vi "Autonomous Independent.vi"   [LabVIEW 2016]
doc: "This VI is called when autonomous begins, and will automatically be terminated when autonomous ends. You can carry out timed or sensor driven robot movement independently without needing to return to the caller."
uses:
  <vilib>/Rock Robotics/WPI/Solenoid/WPI_SolenoidValue.ctl
  <vilib>/Rock Robotics/WPI/DriverStation/WPI_DriverStationAllianceInfo.ctl
  <vilib>/Rock Robotics/Network Tables/NT Read Number.vi
  <vilib>/Rock Robotics/WPI/Solenoid/WPI_SolenoidSetEnum.vi
  Robot Global Data.vi
panel:
  # "Be sure to right-click and choose Data Operations>>Make Current Value default if you want to save the array values with the VI"
types:
  T1 = typedef "WPI_DriverStationAllianceInfo.ctl" = enum16{"Red", "Blue", "Invalid"}
  T2 = typedef "WPI_SolenoidValue.ctl" = enum16{"Off", "On", "Forward", "Reverse"}
  T3 = typedef "WPI_MotorControlDeviceRef.ctl" = cluster{"DeviceStatus":errorcluster, "Type":T4, "PWM":cluster{"PWM Channel":T5, "DeadBand":T6}, "CAN":cluster{"Device Number":u8, "SetOutput VI Ref":variant, "GetOutput VI Ref":variant, "Enable VI Ref":variant, "Disable VI Ref":variant, "Data":variant}, "Invert":bool}
  T4 = typedef "WPI_MotorControlType.ctl" = enum16{"PWM", "CAN"}
  T5 = typedef "FPGA_DIOPWMChannel.ctl" = enum8{"PWM 0", "PWM 1", "PWM 2", "PWM 3", "PWM 4", "PWM 5", "PWM 6", "PWM 7", "PWM 8", "PWM 9", "PWM MXP 0", "PWM MXP 1", "PWM MXP 2", "PWM MXP 3", "PWM MXP 4", "PWM MXP 5", "PWM MXP 6", "PWM MXP 7", "PWM MXP 8", "PWM MXP 9", "Invalid"}
  T6 = typedef "WPI_PWMDeadband.ctl" = cluster{"Name":string, "maxPositivePwm":i32, "minPositivePwm":i32, "centerPwm":i32, "maxNegativePwm":i32, "minNegativePwm":i32, "angularRange":u16}
  T7 = typedef "WPI_SolenoidDevRef.ctl" = cluster{"DevStatus":errorcluster, "Pneumatics Control Module":u8, "Forward Solenoid Channel":T8, "Reverse Solenoid Channel":T8}
  T8 = typedef "WPI_SolenoidChannel.ctl" = enum8{"Solenoid 0", "Solenoid 1", "Solenoid 2", "Solenoid 3", "Solenoid 4", "Solenoid 5", "Solenoid 6", "Solenoid 7", "Invalid"}
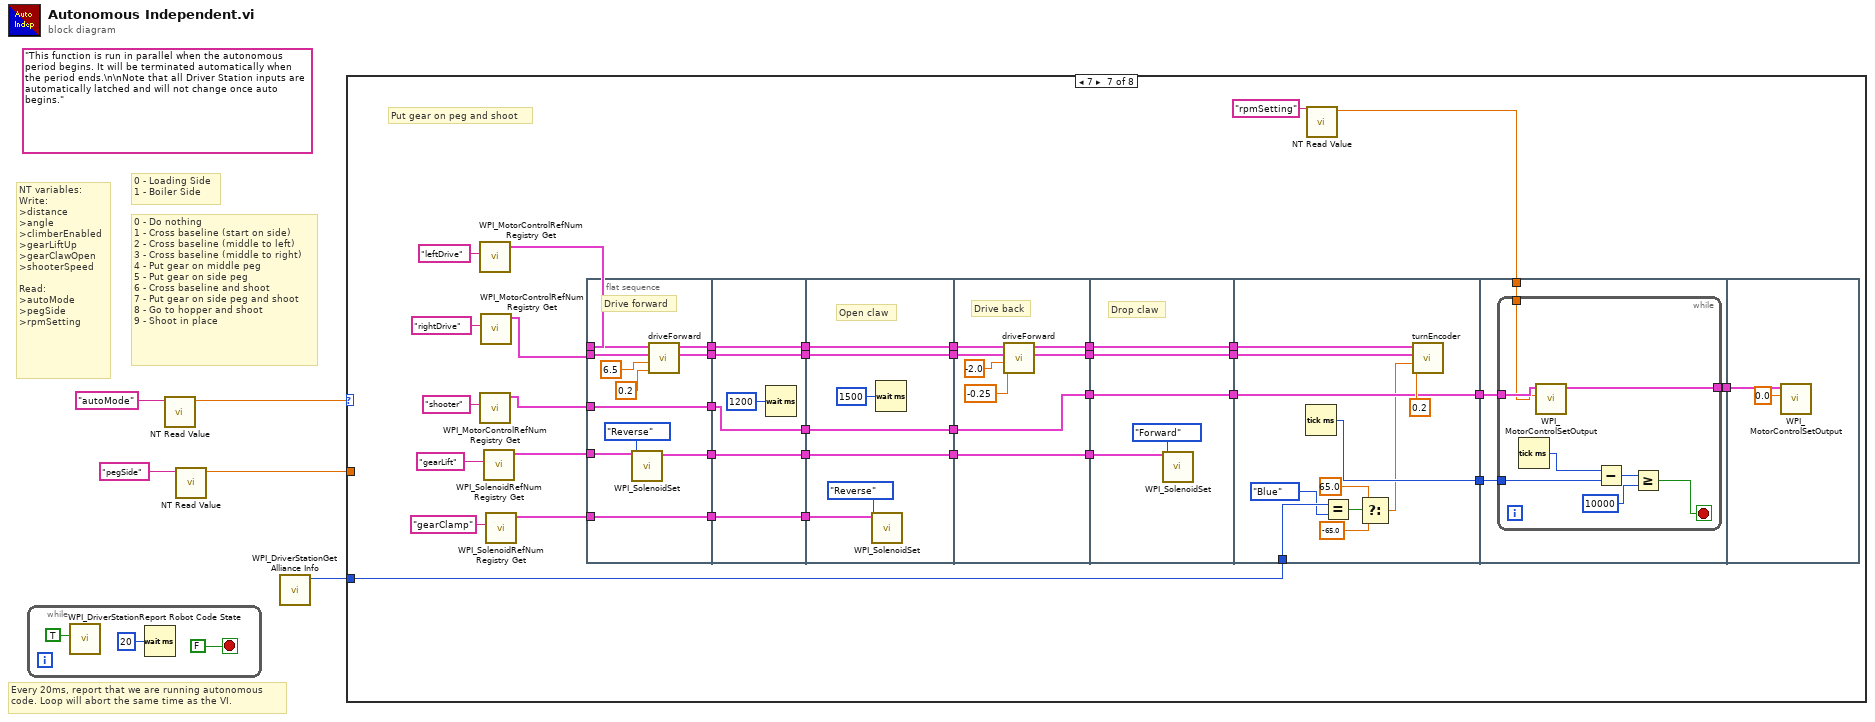
[diagram p0: block diagram]
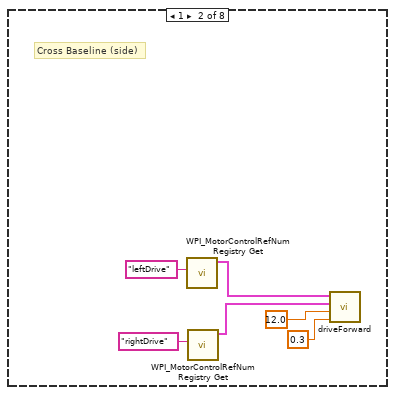
[diagram p3: hidden frame]
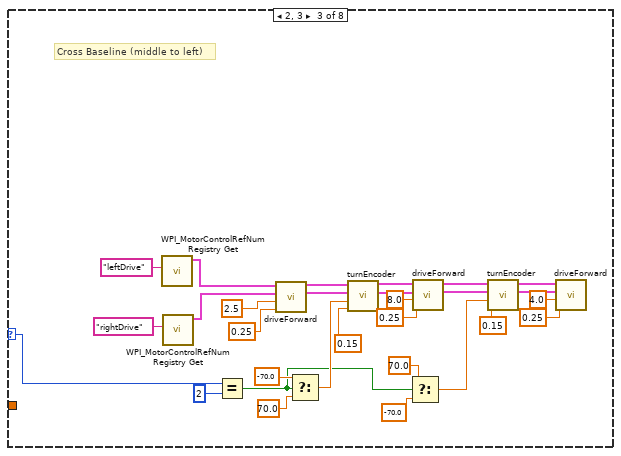
[diagram p4: hidden frame]
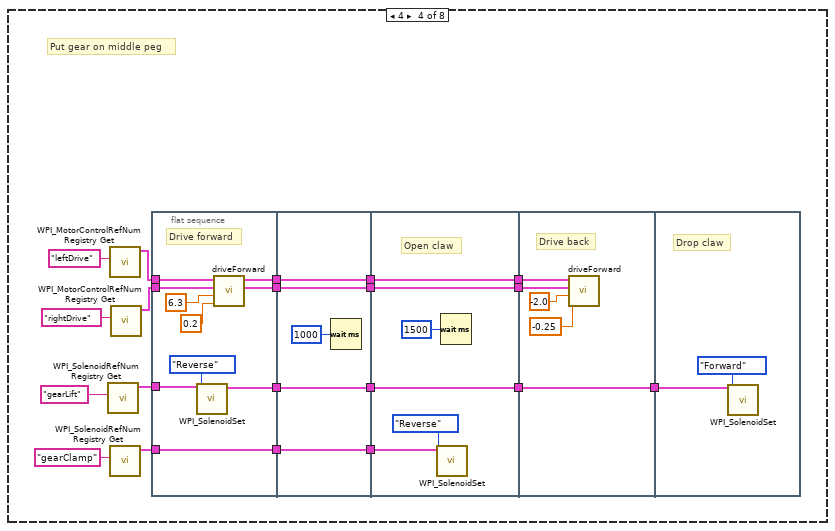
[diagram p5: hidden frame]
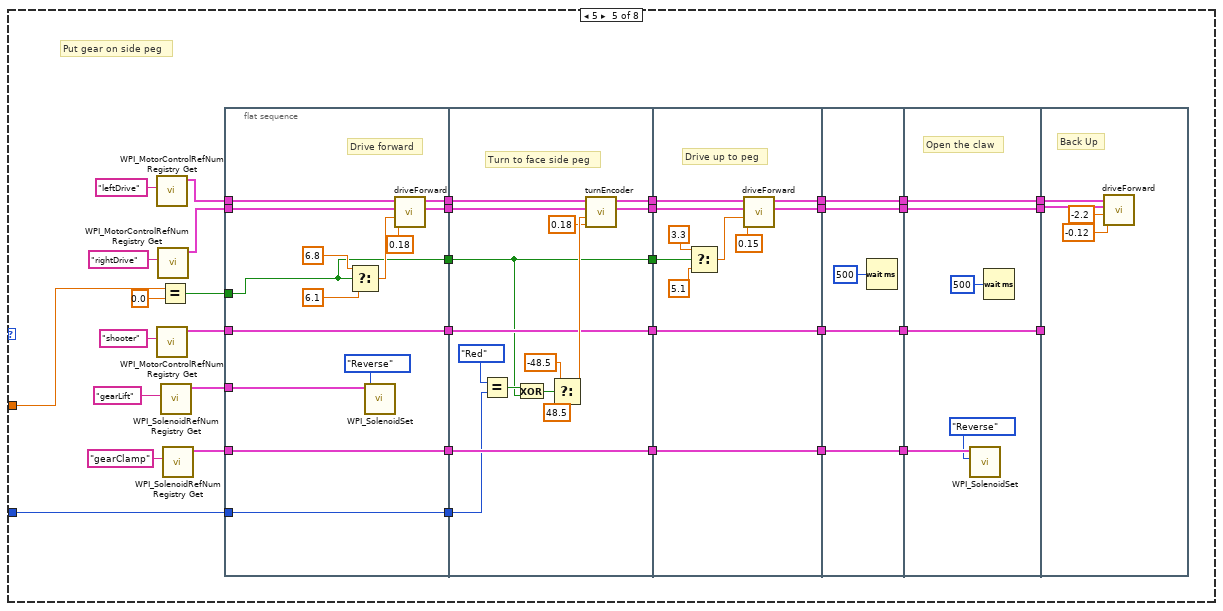
[diagram p6: hidden frame]
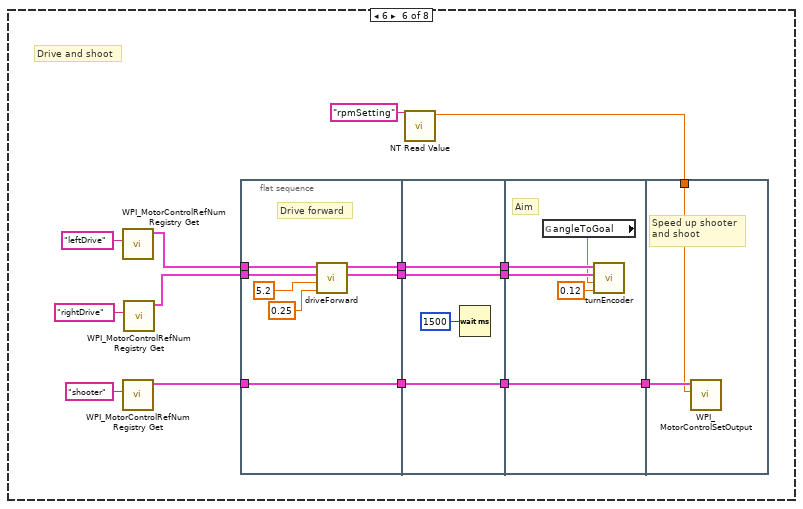
[diagram p7: hidden frame]
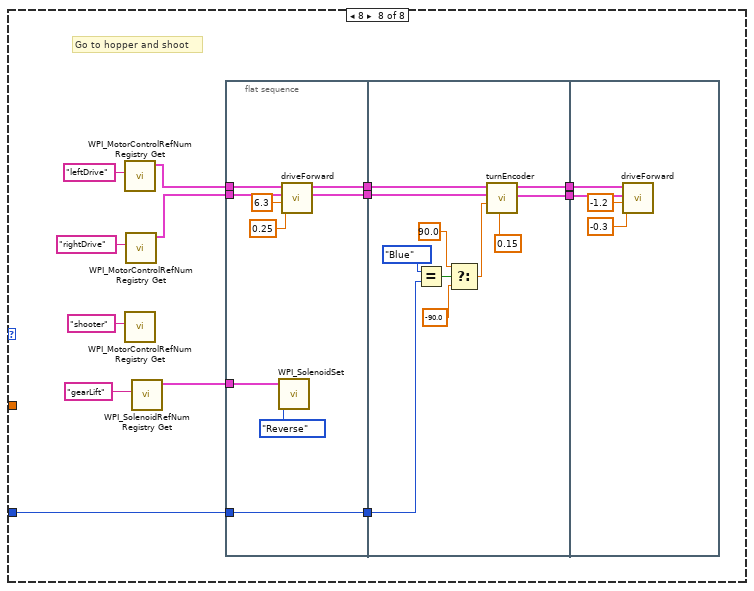
[diagram p8: hidden frame]
diagram:
  (unwired) "This function is run in parallel when the autonomous period begins. It will be terminated automatically when the period ends.\n\nNote that all Driver Station inputs are automatically latched and will not change once auto begins."
  # "0 - Loading Side\n1 - Boiler Side"
  # "NT variables:\nWrite:\n>distance\n>angle\n>climberEnabled\n>gearLiftUp\n>gearClawOpen\n>shooterSpeed\n\nRead:\n>autoMode\n>pegSide\n>rpmSetting"
  # "0 - Do nothing\n1 - Cross baseline (start on side)\n2 - Cross baseline (middle to left)\n3 - Cross baseline (middle to right)\n4 - Put gear on middle peg\n5 - Put gear on side peg\n6 - Cross baseline and shoot\n7 - Put gear on side peg and shoot\n8 - Go to hopper and shoot\n9 - Shoot in place"
  # "Every 20ms, report that we are running autonomous\ncode. Loop will abort the same time as the VI."
  n1 = while {
    stop <- FALSE stop-if-true
    n2 = call <vilib>:"WPI_DriverStationReport Robot Code State.vi"("Autonomous"=TRUE) -> ()  [unwired: 10 in, 1 out]
    n3 = Wait (ms)(milliseconds to wait=u32 20) -> ()  [unwired: 1 out]
  }
  n4 = call-poly <vilib>:"NT Read Value.vi"("Name"="autoMode") -> ("Numeric"=w3:dbl)  [unwired: 9 in, 1 out]
  n5 = call-poly <vilib>:"NT Read Value.vi"("Name"="pegSide") -> ("Numeric"=w1:dbl)  [unwired: 9 in, 1 out]
  n6 = call <vilib>:"WPI_DriverStationGet Alliance Info.vi"() -> ("Alliance"=w4:T1)  [unwired: 11 out]
  n7 = case shown="7" w3 {
    selector: w3 -> [_ _ w20 _ _ _ _ _]
    tunnel: w4 -> [_ _ _ _ w105 _ w216 w318]
    tunnel: w1 -> [_ _ _ _ w103 _ _ _]
    frame 0, Default {
      # "Do nothing"
    }
    frame 1 {
      # "Cross Baseline (side)"
      n8 = call <vilib>:"WPI_MotorControlRefNum Registry Get.vi"("refnum name"="leftDrive") -> ("MotorControlDevRef"=w12:T3)  [unwired: 9 in, 1 out]
      n9 = call <vilib>:"WPI_MotorControlRefNum Registry Get.vi"("refnum name"="rightDrive") -> ("MotorControlDevRef"=w11:T3)  [unwired: 9 in, 1 out]
      n10 = call "driveForward.vi"("speed (%)"=0.3, "distance (ft)"=12.0, "rightMotor"=w11, "leftMotor"=w12) -> ()  [unwired: 6 in, 2 out]
    }
    frame 2, 3 {
      # "Cross Baseline (middle to left)"
      n11 = call <vilib>:"WPI_MotorControlRefNum Registry Get.vi"("refnum name"="leftDrive") -> ("MotorControlDevRef"=w41:T3)  [unwired: 9 in, 1 out]
      n12 = call <vilib>:"WPI_MotorControlRefNum Registry Get.vi"("refnum name"="rightDrive") -> ("MotorControlDevRef"=w40:T3)  [unwired: 9 in, 1 out]
      n13 = Equal?(x=w20, y=2) -> (x = y?=w15:bool)
      n14 = call "driveForward.vi"("speed (%)"=0.25, "distance (ft)"=2.5, "rightMotor"=w40, "leftMotor"=w41) -> ("rightMotor"=w36:T3, "leftMotor"=w37:T3)  [unwired: 6 in]
      n15 = Select(t=-70.0 ("angle (ccw)"), s=w15, f=70.0 ("angle (ccw)")) -> (s? t:f=w22:dbl)
      n16 = call "turnEncoder.vi"("speed (%)"=0.15, "angle (right)"=w22, "rightMotor"=w36, "leftMotor"=w37) -> ("rightMotor"=w33:T3, "leftMotor"=w34:T3)  [unwired: 6 in]
      n17 = Select(t=70.0 ("angle (ccw)"), s=w15, f=-70.0) -> (s? t:f=w17:dbl)
      n18 = call "driveForward.vi"("speed (%)"=0.25, "distance (ft)"=8.0, "rightMotor"=w33, "leftMotor"=w34) -> ("rightMotor"=w29:T3, "leftMotor"=w30:T3)  [unwired: 6 in]
      n19 = call "turnEncoder.vi"("speed (%)"=0.15, "angle (right)"=w17, "rightMotor"=w29, "leftMotor"=w30) -> ("rightMotor"=w26:T3, "leftMotor"=w27:T3)  [unwired: 6 in]
      n20 = call "driveForward.vi"("speed (%)"=0.25, "distance (ft)"=4.0, "rightMotor"=w26, "leftMotor"=w27) -> ()  [unwired: 6 in, 2 out]
    }
    frame 4 {
      # "Put gear on middle peg"
      n21 = call <vilib>:"WPI_SolenoidRefNum Registry Get.vi"("refnum name"="gearLift") -> ("SolenoidDevRef"=w57:T7)  [unwired: 9 in, 1 out]
      n22 = call <vilib>:"WPI_MotorControlRefNum Registry Get.vi"("refnum name"="leftDrive") -> ("MotorControlDevRef"=w61:T3)  [unwired: 9 in, 1 out]
      n23 = call <vilib>:"WPI_SolenoidRefNum Registry Get.vi"("refnum name"="gearClamp") -> ("SolenoidDevRef"=w56:T7)  [unwired: 9 in, 1 out]
      n24 = call <vilib>:"WPI_MotorControlRefNum Registry Get.vi"("refnum name"="rightDrive") -> ("MotorControlDevRef"=w60:T3)  [unwired: 9 in, 1 out]
      n25 = flat-sequence {
        tunnel: w61 -> [w73]
        tunnel: w60 -> [w72]
        tunnel: w57 -> [w69]
        tunnel: [w67] -> w51
        tunnel: w56 -> [w67]
        tunnel: [w66] -> w49
        tunnel: [w65] -> w47
        tunnel: [w64] -> w45
        tunnel: w51 -> [w78]
        tunnel: [w78] -> w50
        tunnel: w49 -> [w77]
        tunnel: [w77] -> w48
        tunnel: w47 -> [w76]
        tunnel: [w76] -> w46
        tunnel: w45 -> [w75]
        tunnel: [w75] -> w44
        tunnel: w50 -> [w84]
        tunnel: [w82] -> w55
        tunnel: w48 -> [w82]
        tunnel: [w81] -> w54
        tunnel: w46 -> [w81]
        tunnel: [w80] -> w52
        tunnel: w44 -> [w80]
        tunnel: w55 -> [w89]
        tunnel: w54 -> [w88]
        tunnel: [w85] -> w53
        tunnel: w52 -> [w85]
        tunnel: w53 -> [w90]
        frame #0 {
          # "Drive forward"
          n26 = call-poly <vilib>:"WPI_SolenoidSet.vi"("Value"=WPI_SolenoidValue."Reverse", "SolenoidDevRef"=w69) -> ("SolenoidDevRef"=w64:T7)  [unwired: 8 in, 1 out]
          n27 = call "driveForward.vi"("speed (%)"=0.2, "distance (ft)"=6.3, "rightMotor"=w72, "leftMotor"=w73) -> ("rightMotor"=w65:T3, "leftMotor"=w66:T3)  [unwired: 6 in]
        }
        frame #1 {
          n28 = Wait (ms)(milliseconds to wait=u32 1000) -> ()  [unwired: 1 out]
        }
        frame #2 {
          # "Open claw"
          n29 = call-poly <vilib>:"WPI_SolenoidSet.vi"("Value"=WPI_SolenoidValue."Reverse", "SolenoidDevRef"=w84) -> ()  [unwired: 8 in, 2 out]
          n30 = Wait (ms)(milliseconds to wait=u32 1500) -> ()  [unwired: 1 out]
        }
        frame #3 {
          # "Drive back"
          n31 = call "driveForward.vi"("speed (%)"=-0.25, "distance (ft)"=-2.0, "rightMotor"=w88, "leftMotor"=w89) -> ()  [unwired: 6 in, 2 out]
        }
        frame #4 {
          # "Drop claw"
          n32 = call-poly <vilib>:"WPI_SolenoidSet.vi"("Value"=WPI_SolenoidValue."Forward", "SolenoidDevRef"=w90) -> ()  [unwired: 8 in, 2 out]
        }
      }
    }
    frame 5 {
      # "Put gear on side peg"
      n33 = call <vilib>:"WPI_MotorControlRefNum Registry Get.vi"("refnum name"="leftDrive") -> ("MotorControlDevRef"=w110:T3)  [unwired: 9 in, 1 out]
      n34 = call <vilib>:"WPI_MotorControlRefNum Registry Get.vi"("refnum name"="shooter") -> ("MotorControlDevRef"=w106:T3)  [unwired: 9 in, 1 out]
      n35 = call <vilib>:"WPI_MotorControlRefNum Registry Get.vi"("refnum name"="rightDrive") -> ("MotorControlDevRef"=w109:T3)  [unwired: 9 in, 1 out]
      n36 = Equal?(x=w103, y=0.0) -> (x = y?=w102:bool)
      n37 = call <vilib>:"WPI_SolenoidRefNum Registry Get.vi"("refnum name"="gearLift") -> ("SolenoidDevRef"=w108:T7)  [unwired: 9 in, 1 out]
      n38 = call <vilib>:"WPI_SolenoidRefNum Registry Get.vi"("refnum name"="gearClamp") -> ("SolenoidDevRef"=w107:T7)  [unwired: 9 in, 1 out]
      n39 = flat-sequence {
        tunnel: w110 -> [w141]
        tunnel: w109 -> [w140]
        tunnel: w105 -> [w138]
        tunnel: [w138] -> w127
        tunnel: [w137] -> w126
        tunnel: [w136] -> w125
        tunnel: w108 -> [w135]
        tunnel: [w133] -> w124
        tunnel: w107 -> [w133]
        tunnel: [w132] -> w123
        tunnel: w106 -> [w132]
        tunnel: w102 -> [w128]
        tunnel: [w128] -> w101
        tunnel: w127 -> [w142]
        tunnel: w126 -> [w153]
        tunnel: w125 -> [w152]
        tunnel: [w149] -> w122
        tunnel: [w148] -> w121
        tunnel: [w147] -> w120
        tunnel: w124 -> [w147]
        tunnel: w123 -> [w146]
        tunnel: [w146] -> w119
        tunnel: w101 -> [w143]
        tunnel: [w143] -> w100
        tunnel: w122 -> [w166]
        tunnel: w121 -> [w165]
        tunnel: [w164] -> w99
        tunnel: w120 -> [w164]
        tunnel: [w163] -> w97
        tunnel: [w162] -> w95
        tunnel: [w161] -> w93
        tunnel: w119 -> [w161]
        tunnel: w100 -> [w158]
        tunnel: w99 -> [w172]
        tunnel: [w172] -> w98
        tunnel: w97 -> [w171]
        tunnel: [w171] -> w96
        tunnel: w95 -> [w170]
        tunnel: [w170] -> w94
        tunnel: w93 -> [w169]
        tunnel: [w169] -> w92
        tunnel: w98 -> [w178]
        tunnel: [w176] -> w118
        tunnel: w96 -> [w176]
        tunnel: w94 -> [w175]
        tunnel: [w175] -> w117
        tunnel: [w174] -> w116
        tunnel: w92 -> [w174]
        tunnel: w118 -> [w182]
        tunnel: w117 -> [w181]
        tunnel: w116 -> [_]
        frame #0 {
          # "Drive forward"
          n40 = Select(t=6.8 ("distance (ft)"), s=w128, f=6.1) -> (s? t:f=w131:dbl)
          n41 = call-poly <vilib>:"WPI_SolenoidSet.vi"("Value"=WPI_SolenoidValue."Reverse", "SolenoidDevRef"=w135) -> ()  [unwired: 8 in, 2 out]
          n42 = call "driveForward.vi"("speed (%)"=0.18, "distance (ft)"=w131, "rightMotor"=w140, "leftMotor"=w141) -> ("rightMotor"=w136:T3, "leftMotor"=w137:T3)  [unwired: 6 in]
        }
        frame #1 {
          # "Turn to face side peg"
          n43 = Equal?(x=WPI_DriverStationAllianceInfo."Red" ("Alliance"), y=w142) -> (x = y?=w145:bool)
          n44 = Exclusive Or(1:w143, 2:w145) -> (0:w144:bool)
          n45 = Select(t=-48.5, s=w144, f=48.5) -> (s? t:f=w151:dbl)
          n46 = call "turnEncoder.vi"("speed (%)"=0.18, "angle (right)"=w151, "rightMotor"=w152, "leftMotor"=w153) -> ("rightMotor"=w148:T3, "leftMotor"=w149:T3)  [unwired: 6 in]
        }
        frame #2 {
          # "Drive up to peg"
          n47 = Select(t=3.3 ("distance (ft)"), s=w158, f=5.1) -> (s? t:f=w159:dbl)
          n48 = call "driveForward.vi"("speed (%)"=0.15, "distance (ft)"=w159, "rightMotor"=w165, "leftMotor"=w166) -> ("rightMotor"=w162:T3, "leftMotor"=w163:T3)  [unwired: 6 in]
        }
        frame #3 {
          n49 = Wait (ms)(milliseconds to wait=u32 500) -> ()  [unwired: 1 out]
        }
        frame #4 {
          # "Open the claw"
          n50 = call-poly <vilib>:"WPI_SolenoidSet.vi"("Value"=WPI_SolenoidValue."Reverse", "SolenoidDevRef"=w178) -> ()  [unwired: 8 in, 2 out]
          n51 = Wait (ms)(milliseconds to wait=u32 500) -> ()  [unwired: 1 out]
        }
        frame #5 {
          # "Back Up"
          n52 = call "driveForward.vi"("speed (%)"=-0.12, "distance (ft)"=-2.2, "rightMotor"=w181, "leftMotor"=w182) -> ()  [unwired: 6 in, 2 out]
        }
      }
    }
    frame 6 {
      # "Drive and shoot"
      n53 = call <vilib>:"WPI_MotorControlRefNum Registry Get.vi"("refnum name"="leftDrive") -> ("MotorControlDevRef"=w195:T3)  [unwired: 9 in, 1 out]
      n54 = call <vilib>:"WPI_MotorControlRefNum Registry Get.vi"("refnum name"="shooter") -> ("MotorControlDevRef"=w190:T3)  [unwired: 9 in, 1 out]
      n55 = call <vilib>:"WPI_MotorControlRefNum Registry Get.vi"("refnum name"="rightDrive") -> ("MotorControlDevRef"=w194:T3)  [unwired: 9 in, 1 out]
      n56 = flat-sequence {
        tunnel: w195 -> [w204]
        tunnel: w194 -> [w203]
        tunnel: [w200] -> w188
        tunnel: [w199] -> w186
        tunnel: [w198] -> w184
        tunnel: w190 -> [w198]
        tunnel: w188 -> [w208]
        tunnel: [w208] -> w187
        tunnel: w186 -> [w207]
        tunnel: [w207] -> w185
        tunnel: w184 -> [w206]
        tunnel: [w206] -> w183
        tunnel: w187 -> [w213]
        tunnel: w185 -> [w212]
        tunnel: [w209] -> w191
        tunnel: w183 -> [w209]
        tunnel: w191 -> [w215]
        tunnel: w189 -> [w214]
        frame #0 {
          # "Drive forward"
          n57 = call "driveForward.vi"("speed (%)"=0.25, "distance (ft)"=5.2, "rightMotor"=w203, "leftMotor"=w204) -> ("rightMotor"=w199:T3, "leftMotor"=w200:T3)  [unwired: 6 in]
        }
        frame #1 {
          n58 = Wait (ms)(milliseconds to wait=u32 1500) -> ()  [unwired: 1 out]
        }
        frame #2 {
          # "Aim"
          n59 = global read "Robot Global Data.vi" "angleToGoal"() -> (w211:dbl)
          n60 = call "turnEncoder.vi"("speed (%)"=0.12, "angle (right)"=w211, "rightMotor"=w212, "leftMotor"=w213) -> ()  [unwired: 6 in, 2 out]
        }
        frame #3 {
          # "Speed up shooter\nand shoot"
          n61 = call <vilib>:"WPI_MotorControlSetOutput.vi"("Output"=w214, "MotorControlDevRef"=w215) -> ()  [unwired: 7 in, 3 out]
        }
      }
      n62 = call-poly <vilib>:"NT Read Value.vi"("Name"="rpmSetting") -> ("Numeric"=w189:dbl)  [unwired: 9 in, 1 out]
    }
    frame 7 {
      # "Put gear on peg and shoot"
      n63 = call <vilib>:"WPI_MotorControlRefNum Registry Get.vi"("refnum name"="leftDrive") -> ("MotorControlDevRef"=w232:T3)  [unwired: 9 in, 1 out]
      n64 = call <vilib>:"WPI_MotorControlRefNum Registry Get.vi"("refnum name"="shooter") -> ("MotorControlDevRef"=w224:T3)  [unwired: 9 in, 1 out]
      n65 = call <vilib>:"WPI_MotorControlRefNum Registry Get.vi"("refnum name"="rightDrive") -> ("MotorControlDevRef"=w233:T3)  [unwired: 9 in, 1 out]
      n66 = call <vilib>:"WPI_SolenoidRefNum Registry Get.vi"("refnum name"="gearLift") -> ("SolenoidDevRef"=w234:T7)  [unwired: 9 in, 1 out]
      n67 = call <vilib>:"WPI_SolenoidRefNum Registry Get.vi"("refnum name"="gearClamp") -> ("SolenoidDevRef"=w231:T7)  [unwired: 9 in, 1 out]
      n68 = flat-sequence {
        tunnel: w232 -> [w263]
        tunnel: w233 -> [w262]
        tunnel: w234 -> [w259]
        tunnel: [w257] -> w246
        tunnel: w231 -> [w257]
        tunnel: [w256] -> w245
        tunnel: [w255] -> w244
        tunnel: [w254] -> w243
        tunnel: [w253] -> w225
        tunnel: w224 -> [w253]
        tunnel: w246 -> [w269]
        tunnel: [w269] -> w242
        tunnel: w245 -> [w268]
        tunnel: [w268] -> w241
        tunnel: w244 -> [w267]
        tunnel: [w267] -> w240
        tunnel: w243 -> [w266]
        tunnel: [w266] -> w239
        tunnel: [w264] -> w226
        tunnel: w225 -> [w264]
        tunnel: w242 -> [w276]
        tunnel: [w274] -> w238
        tunnel: w241 -> [w274]
        tunnel: [w273] -> w237
        tunnel: w240 -> [w273]
        tunnel: [w272] -> w236
        tunnel: w239 -> [w272]
        tunnel: w226 -> [w270]
        tunnel: [w270] -> w220
        tunnel: w238 -> [w284]
        tunnel: w237 -> [w283]
        tunnel: [w280] -> w235
        tunnel: w236 -> [w280]
        tunnel: [w279] -> w229
        tunnel: [w278] -> w228
        tunnel: [w277] -> w221
        tunnel: w220 -> [w277]
        tunnel: w235 -> [w288]
        tunnel: [w287] -> w230
        tunnel: w229 -> [w287]
        tunnel: w228 -> [w286]
        tunnel: [w286] -> w227
        tunnel: [w285] -> w222
        tunnel: w221 -> [w285]
        tunnel: w230 -> [w300]
        tunnel: w227 -> [w299]
        tunnel: [w297] -> w223
        tunnel: w222 -> [w297]
        tunnel: [w296] -> w218
        tunnel: w216 -> [w295]
        tunnel: w223 -> [w304]
        tunnel: w219 -> [w303]
        tunnel: w218 -> [w302]
        tunnel: [w301] -> w217
        tunnel: w217 -> [w314]
        frame #0 {
          # "Drive forward"
          n69 = call-poly <vilib>:"WPI_SolenoidSet.vi"("Value"=WPI_SolenoidValue."Reverse", "SolenoidDevRef"=w259) -> ("SolenoidDevRef"=w254:T7)  [unwired: 8 in, 1 out]
          n70 = call "driveForward.vi"("speed (%)"=0.2, "distance (ft)"=6.5, "rightMotor"=w262, "leftMotor"=w263) -> ("rightMotor"=w255:T3, "leftMotor"=w256:T3)  [unwired: 6 in]
        }
        frame #1 {
          n71 = Wait (ms)(milliseconds to wait=u32 1200) -> ()  [unwired: 1 out]
        }
        frame #2 {
          # "Open claw"
          n72 = call-poly <vilib>:"WPI_SolenoidSet.vi"("Value"=WPI_SolenoidValue."Reverse", "SolenoidDevRef"=w276) -> ()  [unwired: 8 in, 2 out]
          n73 = Wait (ms)(milliseconds to wait=u32 1500) -> ()  [unwired: 1 out]
        }
        frame #3 {
          # "Drive back"
          n74 = call "driveForward.vi"("speed (%)"=-0.25, "distance (ft)"=-2.0, "rightMotor"=w283, "leftMotor"=w284) -> ("rightMotor"=w278:T3, "leftMotor"=w279:T3)  [unwired: 6 in]
        }
        frame #4 {
          # "Drop claw"
          n75 = call-poly <vilib>:"WPI_SolenoidSet.vi"("Value"=WPI_SolenoidValue."Forward", "SolenoidDevRef"=w288) -> ()  [unwired: 8 in, 2 out]
        }
        frame #5 {
          n76 = Tick Count (ms)() -> (millisecond timer value=w296:u32)
          n77 = Equal?(x=w295, y=WPI_DriverStationAllianceInfo."Blue") -> (x = y?=w293:bool)
          n78 = Select(t=65.0, s=w293, f=-65.0) -> (s? t:f=w290:dbl)
          n79 = call "turnEncoder.vi"("speed (%)"=0.2, "angle (right)"=w290, "rightMotor"=w299, "leftMotor"=w300) -> ()  [unwired: 6 in, 2 out]
        }
        frame #6 {
          n80 = while {
            tunnel: w304 -> [w312]
            tunnel: w303 -> [w311]
            tunnel: w302 -> [w309]
            tunnel: [w305] -> w301
            stop <- w306 stop-if-true
            n81 = Tick Count (ms)() -> (millisecond timer value=w310:u32)
            n82 = call <vilib>:"WPI_MotorControlSetOutput.vi"("Output"=w311, "MotorControlDevRef"=w312) -> ("MotorControlDevRef"=w305:T3)  [unwired: 7 in, 2 out]
            n83 = Subtract(x=w310, y=w309) -> (x-y=w308:u32)
            n84 = Greater Or Equal?(x=w308, y=u32 10000) -> (x >= y?=w306:bool)
          }
        }
        frame #7 {
          n85 = call <vilib>:"WPI_MotorControlSetOutput.vi"("Output"=0.0, "MotorControlDevRef"=w314) -> ()  [unwired: 7 in, 3 out]
        }
      }
      n86 = call-poly <vilib>:"NT Read Value.vi"("Name"="rpmSetting") -> ("Numeric"=w219:dbl)  [unwired: 9 in, 1 out]
    }
    frame 8 {
      # "Go to hopper and shoot"
      n87 = call <vilib>:"WPI_MotorControlRefNum Registry Get.vi"("refnum name"="leftDrive") -> ("MotorControlDevRef"=w322:T3)  [unwired: 9 in, 1 out]
      n88 = call <vilib>:"WPI_MotorControlRefNum Registry Get.vi"("refnum name"="shooter") -> ()  [unwired: 9 in, 2 out]
      n89 = call <vilib>:"WPI_MotorControlRefNum Registry Get.vi"("refnum name"="rightDrive") -> ("MotorControlDevRef"=w321:T3)  [unwired: 9 in, 1 out]
      n90 = call <vilib>:"WPI_SolenoidRefNum Registry Get.vi"("refnum name"="gearLift") -> ("SolenoidDevRef"=w323:T7)  [unwired: 9 in, 1 out]
      n91 = flat-sequence {
        tunnel: w323 -> [w336]
        tunnel: w322 -> [w334]
        tunnel: w321 -> [w333]
        tunnel: [w330] -> w320
        tunnel: [w329] -> w319
        tunnel: w318 -> [w328]
        tunnel: [w328] -> w317
        tunnel: w320 -> [w347]
        tunnel: w319 -> [w346]
        tunnel: w317 -> [w342]
        tunnel: [w338] -> w316
        tunnel: [w337] -> w315
        tunnel: w316 -> [w351]
        tunnel: w315 -> [w350]
        frame #0 {
          n92 = call-poly <vilib>:"WPI_SolenoidSet.vi"("Value"=WPI_SolenoidValue."Reverse", "SolenoidDevRef"=w336) -> ()  [unwired: 8 in, 2 out]
          n93 = call "driveForward.vi"("speed (%)"=0.25, "distance (ft)"=6.3, "rightMotor"=w333, "leftMotor"=w334) -> ("rightMotor"=w329:T3, "leftMotor"=w330:T3)  [unwired: 6 in]
        }
        frame #1 {
          n94 = Equal?(x=WPI_DriverStationAllianceInfo."Blue", y=w342) -> (x = y?=w343:bool)
          n95 = Select(t=90.0 ("angle (right)"), s=w343, f=-90.0 ("angle (right)")) -> (s? t:f=w344:dbl)
          n96 = call "turnEncoder.vi"("speed (%)"=0.15, "angle (right)"=w344, "rightMotor"=w346, "leftMotor"=w347) -> ("rightMotor"=w337:T3, "leftMotor"=w338:T3)  [unwired: 6 in]
        }
        frame #2 {
          n97 = call "driveForward.vi"("speed (%)"=-0.3, "distance (ft)"=-1.2, "rightMotor"=w350, "leftMotor"=w351) -> ()  [unwired: 6 in, 2 out]
        }
      }
    }
  }
